vi "multiplot.vi"() -> ()   [LabVIEW 2018]
panel:
  out "Waveform Graph 3":cluster{dbl, dbl, dbl[]}[](graph)
  in  "Tab Control":enum32{"Page 1", "Page 2"}(tab)
  out "Waveform Chart":cluster{"number: 0 to 1":dbl, dbl}(graph)
  out "Waveform Graph":dbl[](graph)
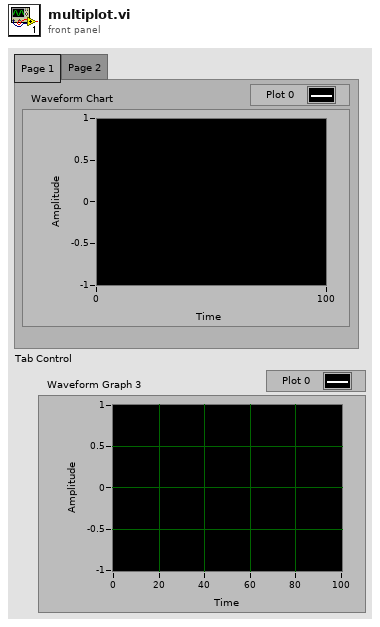
[diagram p1: front panel]
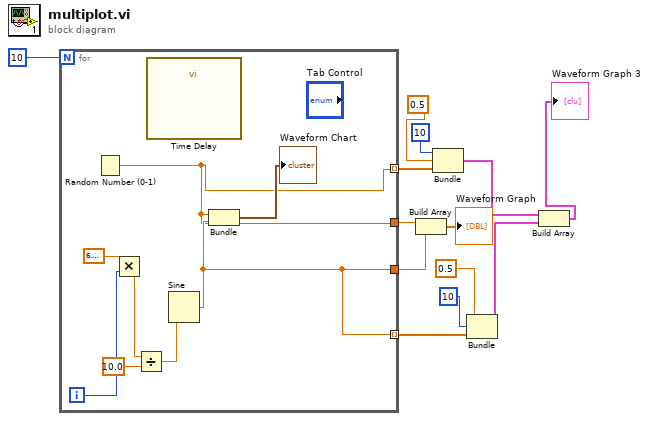
[diagram p0: block diagram]
diagram:
  n1 = for {
    N: 10 -> [_]
    tunnel: [w16] -> w8
    tunnel: [w15] -> w10
    tunnel: [w15] -> w3 mode=indexing
    tunnel: [w16] -> w2 mode=indexing
    i -> [w21]
    n2 = Random Number (0-1)() -> (number: 0 to 1=w15:dbl)
    n3 = Multiply(x=6.283185307179586, y=w21) -> (x*y=w19:dbl)
    n4 = Divide(x=w19, y=10.0) -> (x/y=w18:dbl)
    n5 = call "Time Delay"() -> ()  [unwired: 11 in, 1 out]
    n6 = Sine(x=w18) -> (sin(x)=w16:dbl)
    n7 = Bundle("number: 0 to 1"=w15, w16) -> (→"Waveform Chart":cluster{"number: 0 to 1":dbl, dbl})  [unwired: 1 in]
  }
  n8 = Build Array(w10, w8) -> (→"Waveform Graph":dbl[])
  n9 = Bundle(10, 0.5, w3) -> (w4:cluster{i32, dbl, dbl[]})  [unwired: 1 in]
  n10 = Bundle(0.5, 10, w2) -> (w5:cluster{dbl, i32, dbl[]})  [unwired: 1 in]
  n11 = Build Array(w4, w5) -> (→"Waveform Graph 3":cluster{dbl, dbl, dbl[]}[])
